vi "test BC Only.vi"(8 "error in":errorcluster, 11 "TestCase in":refnum<class "Create Execution Unit.lvclass">) -> (0 "error out":errorcluster, 3 "TestCase out":refnum<class "Create Execution Unit.lvclass">)   [LabVIEW 2020, in "Create Execution Unit.lvclass"]
uses:
  Create Execution Unit.lvclass
  C:/Users/nitest/Desktop/Git 2020/niveristand-custom-device-testing-tools/VeriStandScriptingTestCase/VeriStandScriptingTestCase.lvclass
  niveristand-custom-device-testing-tools/VeriStandScriptingTestCase/VeriStandScriptingTestCase.lvclass/VeriStandScriptingTestCase.ctl
  niveristand-custom-device-testing-tools/VeriStandScriptingTestCase/Read Target.vi
  NationalInstruments.VeriStand.SystemDefinitionAPI
  <vilib>/addons/_JKI Toolkits/VI Tester/TestCase.llb/TestCase.lvclass
  Shared/Address.ctl
  C:/Program Files (x86)/National Instruments/LabVIEW 2020/vi.lib/addons/_JKI Toolkits/VI Tester/TestCase.llb/TestCase.lvclass
  C:/Users/nitest/Desktop/Git 2020/niveristand-aim-milStd1553-custom-device/Source/Custom Device Support/Tests/Unit/Create Execution Unit/Create Execution Unit.lvclass
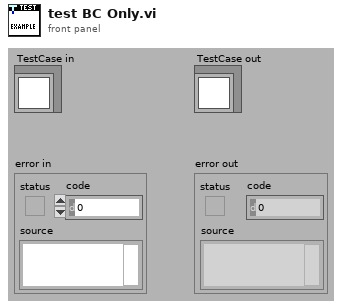
[diagram p1: front panel]
types:
  T1 = typedef "Address.ctl" = u16
  T2 = cluster{"Rx Channel Counts":cluster{"Incoming":i32, "Outgoing":i32, "ReadWrite":i32}, "Rx Message Count":i32, "Tx Acyclic Channel Counts":cluster{"Incoming":i32, "Outgoing":i32, "ReadWrite":i32}, "Triggerable Frames Count":i32, "Tx Channel Counts":cluster{"Incoming":i32, "Outgoing":i32, "ReadWrite":i32}, "Transmitted Message Count":i32, "Expected terminals":T1[], "Expected messages":i32}
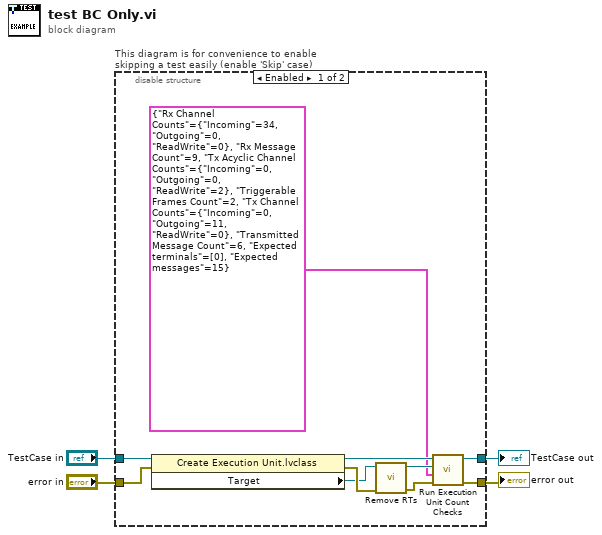
[diagram p0: block diagram]
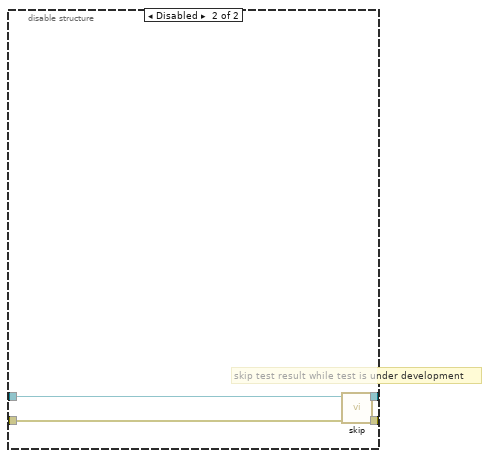
[diagram p2: hidden frame]
diagram:
  n1 = disable-structure "This diagram is for convenience to enable skipping a test easily (enable 'Skip' case)" shown="Enabled" {
    disable-tunnel: "TestCase in" -> [w13 w18]
    disable-tunnel: [w6 w16] -> w1
    disable-tunnel: [w7 w17] -> w3
    disable-tunnel: "error in" -> [w14 w15]
    frame Enabled {
      n2 = property class="Create Execution Unit.lvclass"(reference=w13, error in=w14) -> (reference out=w9:refnum<class "Create Execution Unit.lvclass">, error out=w12:errorcluster, "Target"=w8:refnum<k24>)
      n3 = call "Remove RTs.vi"("error in"=w12, "Target in"=w8) -> ("error out"=w10:errorcluster, "Target out"=w11:refnum<k24>)  [unwired: 8 in]
      n4 = call "Run Execution Unit Count Checks.vi"("error in"=w10, "Test Configuration"=T2 {"Rx Channel Counts"={"Incoming"=34, "Outgoing"=0, "ReadWrite"=0}, "Rx Message Count"=9, "Tx Acyclic Channel Counts"={"Incoming"=0, "Outgoing"=0, "ReadWrite"=2}, "Triggerable Frames Count"=2, "Tx Channel Counts"={"Incoming"=0, "Outgoing"=11, "ReadWrite"=0}, "Transmitted Message Count"=6, "Expected terminals"=[0], "Expected messages"=15}, "Target in"=w11, "Create Execution Unit in"=w9) -> ("error out"=w7:errorcluster, "Create Execution Unit out"=w6:refnum<class "Create Execution Unit.lvclass">)  [unwired: 6 in]
    }
    frame Disabled {
      # "skip test result while test is under development"
      n5 = call <vilib>:"skip.vi"("error in (no error)"=w15, "TestCase in"=w18) -> ("error out"=w17:errorcluster, "TestCase out"=w16:refnum<class "Create Execution Unit.lvclass">)  [unwired: 8 in]
    }
  }
  "error out" <- w3
  "TestCase out" <- w1
